vi "2b_Datalog read.vi"() -> ()   [LabVIEW 2010]
panel:
  in  "stop":bool
  in  "offset (in records) (0)":i64
  out "# of records":i64
  out "Waveform Graph":dbl[][](graph)
  out "Header":string
  out "Record ID":string
  in  "Cluster":T1
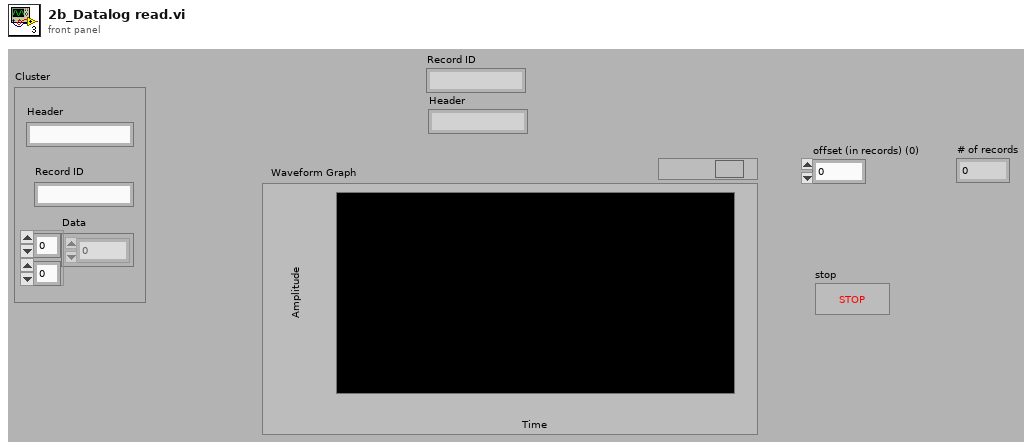
[diagram p1: front panel]
types:
  T1 = cluster{"Data":dbl[][], "Header":string, "Record ID":string}
  T2 = enum16{"open", "replace", "create", "open or create", "replace or create", "replace or create with confirmation"}
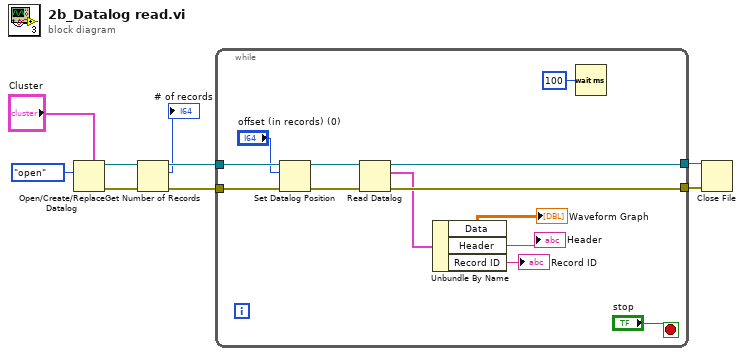
[diagram p0: block diagram]
diagram:
  n1 = Open/Create/Replace Datalog(5:"Cluster", 10:T2."open" ("operation (0:open)")) -> (0:w4:errorcluster, 3:w5:refnum<k1>)  [unwired: 4 in, 1 out]
  n2 = Get Number of Records(4:w4, 7:w5) -> (0:w3:errorcluster, 2:→"# of records":i64, 3:w2:refnum<k1>)
  n3 = while {
    tunnel: [w21] -> w8
    tunnel: [w20] -> w7
    tunnel: w3 -> [w15]
    tunnel: w2 -> [w14]
    stop <- "stop" stop-if-true
    n4 = Set Datalog Position(4:w15, 6:"offset (in records) (0)", 7:w14) -> (0:w12:errorcluster, 3:w13:refnum<k1>)  [unwired: 1 in]
    n5 = Read Datalog(4:w12, 7:w13) -> (0:w21:errorcluster, 2:w19:T1, 3:w20:refnum<k1>)  [unwired: 1 in]
    n6 = Unbundle By Name(w19) -> ("Data"=→"Waveform Graph":dbl[][], "Header"=→"Header":string, "Record ID"=→"Record ID":string)
    n7 = Wait (ms)(milliseconds to wait=u32 100) -> ()  [unwired: 1 out]
  }
  n8 = Close File(refnum=w7, error in=w8) -> ()  [unwired: 2 out]
